vi "Overrid Dynamic Dispatch VIs.vi"(8 "error in (no error)":errorcluster, 11 "Mock Class Generator in":refnum<class "Mock Class Generator.lvclass">) -> (0 "error out":errorcluster, 3 "Mock Class Generator out":refnum<class "Mock Class Generator.lvclass">)   [LabVIEW 2020, in "Mock Class Generator.lvclass"]
uses:
  Mock Class Generator.lvclass
  Mock Class Generator.lvclass/Mock Class Generator.ctl
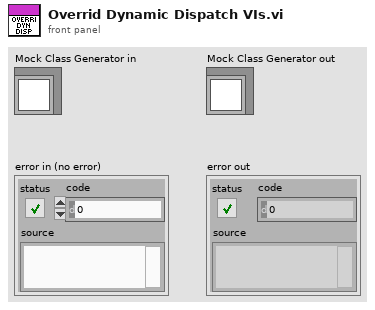
[diagram p1: front panel]
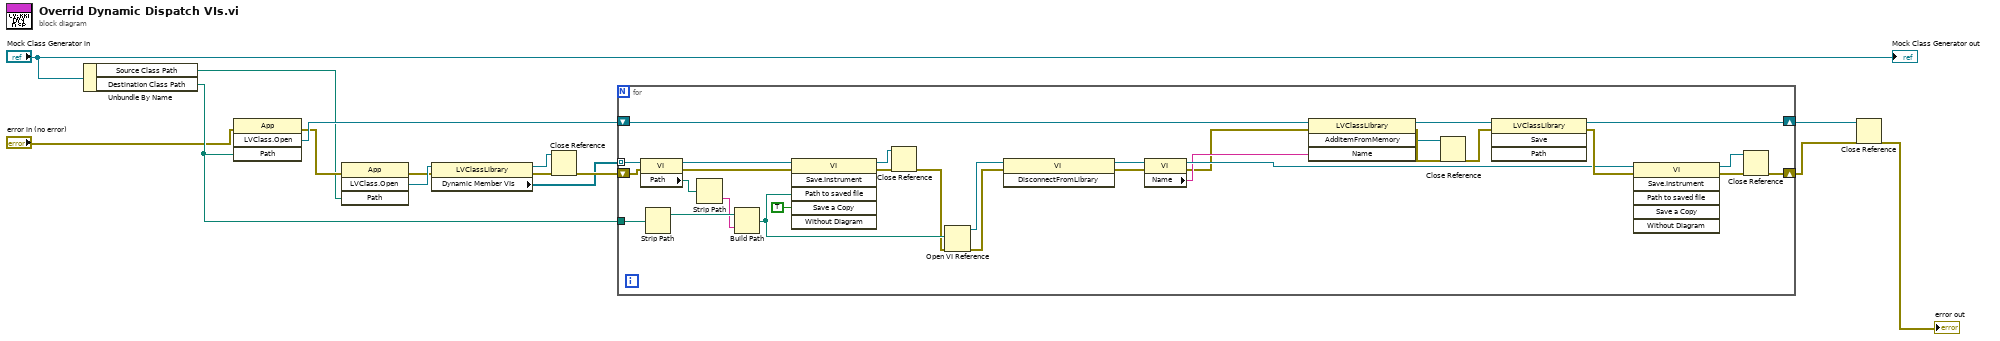
[diagram p0: block diagram]
diagram:
  n1 = Unbundle By Name("Mock Class Generator in") -> ("Source Class Path"=w10:path, "Destination Class Path"=w14:path)
  n2 = invoke class="App" method="LVClass.Open"(error in="error in (no error)", "Path"=w14) -> (error out=w12:errorcluster, "LVClass.Open"=w13:refnum<vi>)  [unwired: 2 in, 2 out]
  n3 = invoke class="App" method="LVClass.Open"(error in=w12, "Path"=w10) -> (error out=w8:errorcluster, "LVClass.Open"=w9:refnum<vi>)  [unwired: 2 in, 2 out]
  n4 = property class="LVClassLibrary"(reference=w9, error in=w8) -> (reference out=w2:refnum<vi>, error out=w3:errorcluster, "Dynamic Member VIs"=w4:refnum<vi>[])
  n5 = Close Reference(reference=w2, error in (no error)=w3) -> (error out=w5:errorcluster)
  n6 = for {
    tunnel: w4 -> [w45] mode=indexing
    shift-right: [w32] -> w6
    shift-left: w5 -> [w39]
    shift-right: [w30] -> w7
    shift-left: w13 -> [w37]
    tunnel: w14 -> [w16]
    n7 = property class="VI"(reference=w45, error in=w39) -> (reference out=w40:refnum<vi>, error out=w38:errorcluster, "Path"=w44:path)
    n8 = Strip Path(path=w16) -> (stripped path=w43:path)  [unwired: 1 out]
    n9 = Strip Path(path=w44) -> (name=w42:string)  [unwired: 1 out]
    n10 = Build Path(base path=w43, name or relative path=w42) -> (appended path=w20:path)
    n11 = invoke class="VI" method="Save.Instrument"(reference=w40, error in=w38, "Path to saved file"=w20, "Save a Copy"=TRUE) -> (reference out=w21:refnum<vi>, error out=w24:errorcluster)  [unwired: 2 in, 4 out]
    n12 = Close Reference(reference=w21, error in (no error)=w24) -> (error out=w19:errorcluster)
    n13 = Open VI Reference(vi path=w20, error in (no error)=w19) -> (vi reference=w18:refnum<vi>, error out=w17:errorcluster)  [unwired: 4 in]
    n14 = invoke class="VI" method="DisconnectFromLibrary"(reference=w18, error in=w17) -> (reference out=w22:refnum<vi>, error out=w23:errorcluster)  [unwired: 1 in, 1 out]
    n15 = property class="VI"(reference=w22, error in=w23) -> (reference out=w27:refnum<vi>, error out=w25:errorcluster, "Name"=w26:string)
    n16 = invoke class="LVClassLibrary" method="AddItemFromMemory"(reference=w37, error in=w25, "Name"=w26) -> (reference out=w31:refnum<vi>, error out=w36:errorcluster, "AddItemFromMemory"=w35:refnum<vi>)  [unwired: 1 in, 1 out]
    n17 = Close Reference(reference=w35, error in (no error)=w36) -> (error out=w29:errorcluster)
    n18 = invoke class="LVClassLibrary" method="Save"(reference=w31, error in=w29) -> (reference out=w30:refnum<vi>, error out=w28:errorcluster)  [unwired: 2 in, 2 out]
    n19 = invoke class="VI" method="Save.Instrument"(reference=w27, error in=w28) -> (reference out=w34:refnum<vi>, error out=w33:errorcluster)  [unwired: 4 in, 4 out]
    n20 = Close Reference(reference=w34, error in (no error)=w33) -> (error out=w32:errorcluster)
  }
  n21 = Close Reference(reference=w7, error in (no error)=w6) -> (error out=→"error out":errorcluster)
  "Mock Class Generator out" <- "Mock Class Generator in"
